vi "Create ModuleA.vi"(5 "ConfigManager":refnum<class "ConfigManager.lvclass">, 7 "Shared Resource (F)":bool, 8 "error in (no error)":errorcluster, 10 "Subsystem Name (optional)":string, 11 "ModuleA in":refnum<class "ModuleA.lvclass">) -> (0 "error out":errorcluster, 2 "SMO name":string, 3 "ModuleA out":refnum<class "ModuleA.lvclass">)   [LabVIEW 2014]
uses:
  ModuleA.lvclass
  <vilib>/LabVIEW Open Source Project/Configuration Manager/Manager/ConfigManager.lvclass
  <vilib>/LabVIEW Open Source Project/Configuration Manager/Manager/Decompose KVPs.vi
  <vilib>/LabVIEW Open Source Project/Configuration Manager/Manager/Write.vi
  <vilib>/JKI/JKI SMO/SMO/SMO.lvclass
  <vilib>/LabVIEW Open Source Project/Configuration Manager/Cache/ConfigManager.Cache.lvclass
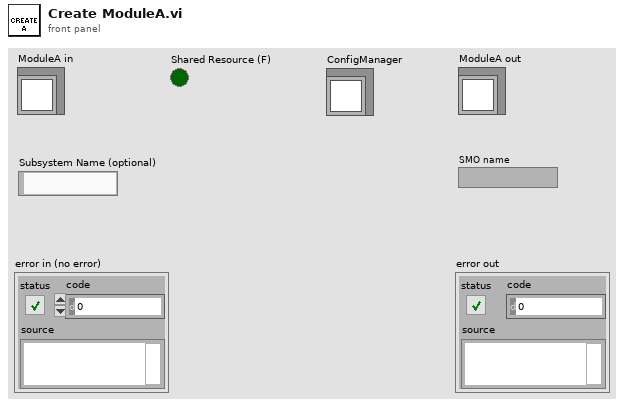
[diagram p1: front panel]
types:
  T1 = typedef "ModuleA.lvclass/Configuration - cluster.ctl" = cluster{"Boolean":bool, "Numeric":dbl, "Numeric 2":dbl, "String":string}
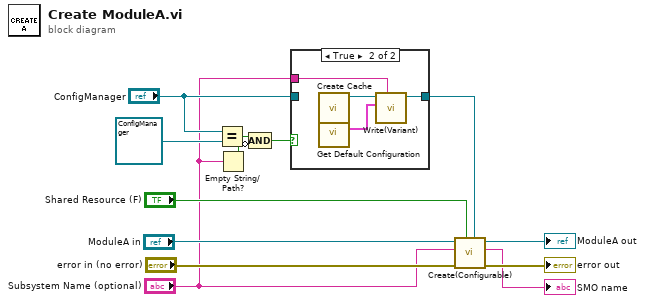
[diagram p0: block diagram]
diagram:
  n1 = Equal?(x="ConfigManager", y=refnum<class "ConfigManager.lvclass"> refnum ("ConfigManager")) -> (x = y?=w4:bool)
  n2 = Empty String/Path?(string/path="Subsystem Name (optional)") -> (empty?=w2:bool)
  n3 = Compound Arithmetic op=AND(w4, invert w2) -> (w3:bool)
  n4 = case shown="True" w3 {
    tunnel: [w14 w17] -> w9
    tunnel: "ConfigManager" -> [w14 _]
    tunnel: "Subsystem Name (optional)" -> [_ w15]
    frame False {
    }
    frame True {
      n5 = call <vilib>:"Create Cache.vi"() -> ("ConfigManager.Cache"=w18:refnum<class "ConfigManager.Cache.lvclass">)  [unwired: 11 in]
      n6 = call "Get Default Configuration.vi"() -> ("Configuration"=w16:T1)  [unwired: 11 in]
      n7 = call <vilib>:"Write(Variant).vi"("Qualified Name"=w15, "value"=w16, "ConfigManager in"=w18) -> ("ConfigManager out"=w17:refnum<class "ConfigManager.Cache.lvclass">)  [unwired: 6 in, 2 out]
    }
  }
  n8 = call <vilib>:"Create(Configurable).vi"("ConfigManager"=w9, "Shared Resource (F)"="Shared Resource (F)", "error in (no error)"="error in (no error)", "Subsystem Name (optional)"="Subsystem Name (optional)", "SMO"="ModuleA in") -> ("error out"=→"error out":errorcluster, "SMO name"=→"SMO name":string, "SMO out"=→"ModuleA out":refnum<class "ModuleA.lvclass">)  [unwired: 4 in]
